vi "DAQ_DO_WF.vi"(8 "error in":errorcluster caption="entrée d'erreur", 10 "Readout time (s)":dbl=0.1, 11 "Exposure time (s)":dbl=0.1) -> (0 "error out":errorcluster caption="sortie d'erreur", 1 "Graphe":waveform(i16)(graph), 2 "Dimension":u32, 3 "DO table":bool[](array[boolean]))   [LabVIEW 2025]
uses:
  Controls/TypeDef_FGV.ctl
  FGV/FGV_DO_Table.vi
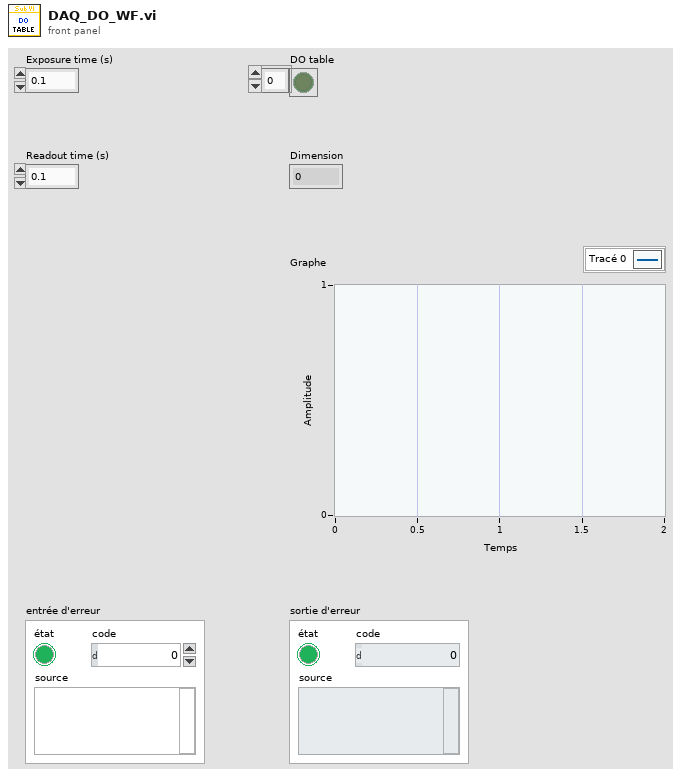
[diagram p1: front panel]
types:
  T1 = typedef "TypeDef_FGV.ctl" = enum16{"Initialize", "Write", "Read"}
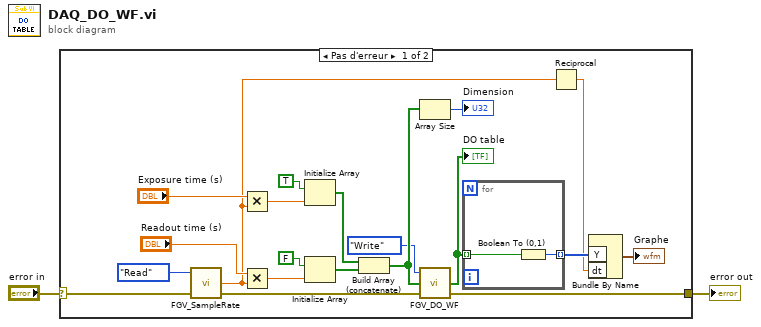
[diagram p0: block diagram]
diagram:
  n1 = case shown="Pas d'erreur" "error in" {
    selector: "error in" -> [w21 w25]
    tunnel: [w9 w25] -> w1
    frame No Error {
      n2 = call "FGV_SampleRate.vi"("error in"=w21, "Action"=TypeDef_FGV."Read") -> ("error out"=w11:errorcluster, "CO task"=w5:dbl)  [unwired: 2 in]
      n3 = Multiply(x="Exposure time (s)", y=w5) -> (x*y=w22:dbl)
      n4 = Multiply(x="Readout time (s)", y=w5) -> (x*y=w16:dbl)
      n5 = Initialize Array(TRUE, w22) -> (w15:bool[])
      n6 = Initialize Array(FALSE, w16) -> (w14:bool[])
      n7 = Build Array (concatenate)(w15, w14) -> (w10:bool[])
      n8 = Array Size(array=w10) -> (size(s)=→"Dimension":i32)
      n9 = call "FGV_DO_WF.vi"("error in"=w11, "DO table"=w10, "Action"=TypeDef_FGV."Write") -> ("error out"=w9:errorcluster, "DO table"=w7:bool[])  [unwired: 1 in]
      "DO table" <- w7
      n10 = for {
        tunnel: w7 -> [w24] mode=indexing
        tunnel: [w23] -> w6 mode=indexing
        n11 = Boolean To (0,1)(Boolean=w24) -> (0, 1=w23:i16)
      }
      n12 = Reciprocal(x=w5) -> (1/x=w4:dbl)
      n13 = Bundle By Name("Y"=w6, "dt"=w4) -> (→"Graphe":waveform(i16))  [unwired: 1 in]
    }
    frame Error {
    }
  }
  "error out" <- w1
